vi "AlliGator Move Cursor n to Reference n.vi"(8 "Error In":errorcluster, 10 "Reference n":i32, 11 "Phasor Graph Refnum":refnum<vi>) -> (0 "Error Out":errorcluster, 2 "Reference Idx":i32, 3 "Reference Phasor":T1)   [LabVIEW 2021, in "AlliGator Phasor Graph.lvlib"]
doc: "Moves cursor to the specified reference (if it exists)."
uses:
  AlliGator Phasor Graph.lvlib
  Phasor/Phasor (g, s).ctl
  AlliGator Phasor Ratio.lvlib
  Graphs/Graphs.lvlib
  Phasor/Phasor.lvlib
panel:
  # "see the AlliGator License on the block diagram (Ctrl+E or Window:Show Block Diagram)"
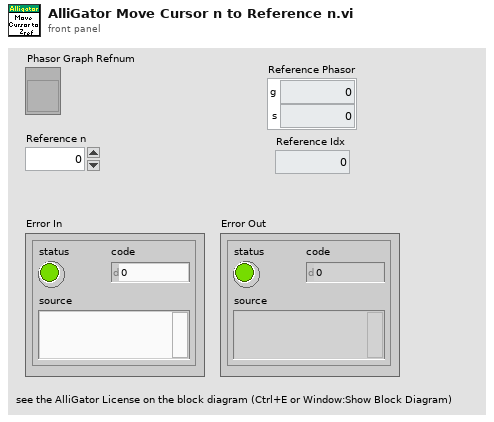
[diagram p1: front panel]
types:
  T1 = typedef "Phasor.lvlib/Phasor (g, s).ctl" = cluster{"g":dbl, "s":dbl}
  T2 = enum16{"use last cursor mode", "free", "single-plot", "multiplot"}
  T3 = typedef "LVCursorListTypeDef.ctl" = cluster{"Name":string, "Color":u32, "Style":u8, "Point Style":u8, "Name Visible":bool, "Allow Drag":bool, "Cursor Mode":u32, "Plot":i32, "Index":i32, "Position":cluster{"X":dbl, "Y":dbl}, "X Scale":u32, "Y Scale":u32, "Watch Plots":i32[], "Watch All Plots":bool, "Plot Area":i32, "Label Offset":cluster{"X":dbl, "Y":dbl}}[]
  T4 = cluster{"Name":string, "Color":u32, "Style":u8, "Point Style":u8, "Name Visible":bool, "Allow Drag":bool, "Cursor Mode":u32, "Plot":i32, "Index":i32, "Position":cluster{"X":dbl, "Y":dbl}, "X Scale":u32, "Y Scale":u32, "Watch Plots":i32[], "Watch All Plots":bool, "Plot Area":i32, "Label Offset":cluster{"X":dbl, "Y":dbl}}
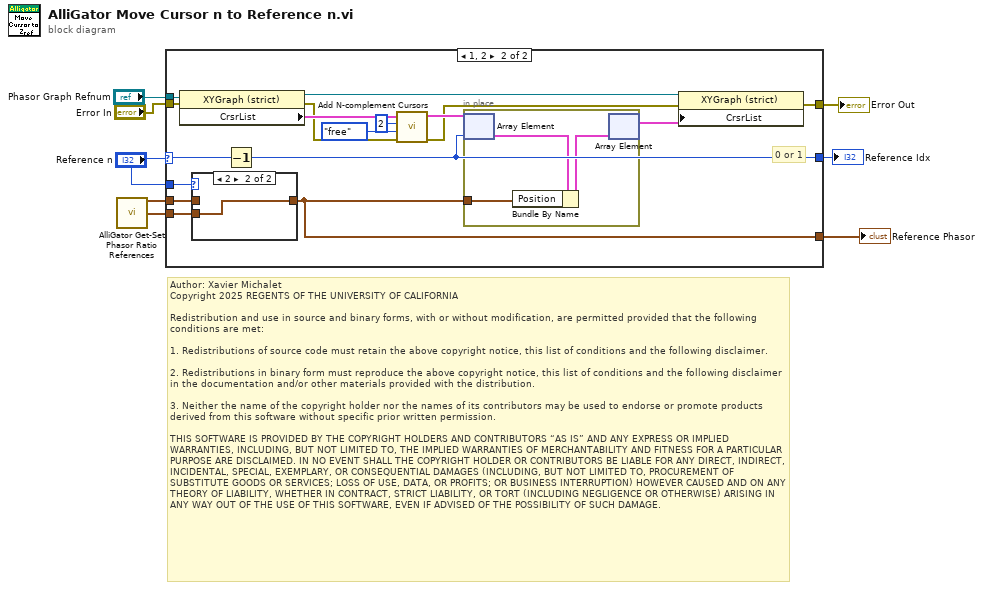
[diagram p0: block diagram]
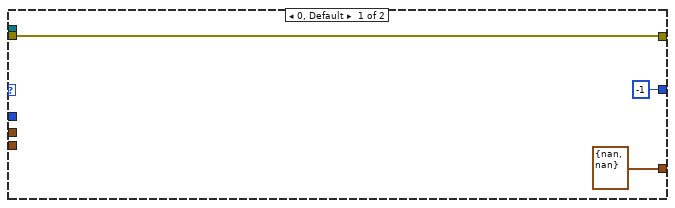
[diagram p2: hidden frame]
diagram:
  # "Author: Xavier Michalet\nCopyright 2025 REGENTS OF THE UNIVERSITY OF CALIFORNIA\n\nRedistribution and use in source and binary forms, with or without modification, are permitted provided that the following conditions are met:\n\n1. Redistributions of source code must retain the above copyright notice, this list of conditions and the following disclaimer.\n\n2. Redistributions in binary form must reproduce the above copyright notice, this list of conditions and the following disclaimer in the documentation and/or other materials provided with the distribution.\n\n3. Neither the name of the copyright holder nor the names of its contributors may be used to endorse or promote products derived from this software without specific prior written permission.\n\nTHIS SOFTWARE IS PROVIDED BY THE COPYRIGHT HOLDERS AND CONTRIBUTORS “AS IS” AND ANY EXPRESS OR IMPLIED WARRANTIES, INCLUDING, BUT NOT LIMITED TO, THE IMPLIED WARRANTIES OF MERCHANTABILITY AND FITNESS FOR A PARTICULAR PURPOSE ARE DISCLAIMED. IN NO EVENT SHALL THE COPYRIGHT HOLDER OR CONTRIBUTORS BE LIABLE FOR ANY DIRECT, INDIRECT, INCIDENTAL, SPECIAL, EXEMPLARY, OR CONSEQUENTIAL DAMAGES (INCLUDING, BUT NOT LIMITED TO, PROCUREMENT OF SUBSTITUTE GOODS OR SERVICES; LOSS OF USE, DATA, OR PROFITS; OR BUSINESS INTERRUPTION) HOWEVER CAUSED AND ON ANY THEORY OF LIABILITY, WHETHER IN CONTRACT, STRICT LIABILITY, OR TORT (INCLUDING NEGLIGENCE OR OTHERWISE) ARISING IN ANY WAY OUT OF THE USE OF THIS SOFTWARE, EVEN IF ADVISED OF THE POSSIBILITY OF SUCH DAMAGE."
  n1 = call "AlliGator Get-Set Phasor Ratio References.vi"() -> ("Reference Phasor 1"=w8:T1, "Reference Phasor 2"=w7:T1)  [unwired: 8 in, 6 out]
  n2 = case shown="1, 2" "Reference n" {
    tunnel: w8 -> [_ w27]
    tunnel: w7 -> [_ w26]
    tunnel: "Phasor Graph Refnum" -> [_ w25]
    tunnel: "Error In" -> [w11 w24]
    tunnel: "Reference n" -> [_ w19]
    tunnel: [w11 w14] -> w4
    tunnel: [T1 {"g"=nan, "s"=nan} ("Reference Phasor 2") w13] -> w2
    tunnel: [-1 w12] -> w1
    frame 0, Default {
    }
    frame 1, 2 {
      # "0 or 1"
      n3 = property class="XYGraph (strict)"(reference=w25, error in=w24) -> (reference out=w17:refnum<vi>, error out=w21:errorcluster, "CrsrList"=w23:T3)
      n4 = case shown="2" w19 {
        tunnel: w27 -> [w31 _]
        tunnel: [w31 w32] -> w13
        tunnel: w26 -> [_ w32]
        frame 1, Default {
        }
        frame 2 {
        }
      }
      n5 = Decrement(x=w19) -> (x-1=w12:i32)
      n6 = call "Add N-complement Cursors.vi"("Error In"=w21, "Cursor Mode"=T2."free", "Total Cursor Number"=2, "CrsrList in"=w23) -> ("Error Out"=w16:errorcluster, "CrsrList out"=w18:T3)  [unwired: 6 in]
      n7 = in-place {
        in-place-border: w13 -> [w28]
        n8 = in-place-array #1(w18, w12) -> (w30:T4)
        n9 = Bundle By Name(cluster=w30, "Position"=w28) -> (w29:T4)
        n10 = in-place-array #1(w29) -> (w15:T3)  [unwired: 1 out]
      }
      n11 = property class="XYGraph (strict)"(reference=w17, error in=w16, "CrsrList"=w15) -> (error out=w14:errorcluster)  [unwired: 1 out]
    }
  }
  "Error Out" <- w4
  "Reference Phasor" <- w2
  "Reference Idx" <- w1
